vi "DigitalRead.vi"() -> ()   [LabVIEW 2014]
panel:
  in  "Port":u8
  in  "Info In":cluster{"Numeric":u8}
  out "Info Out":cluster{"Numeric":u8}
  out "Reply":string
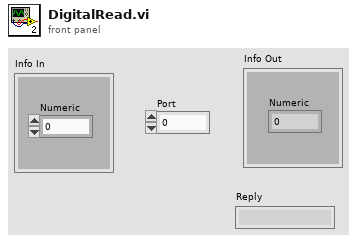
[diagram p1: front panel]
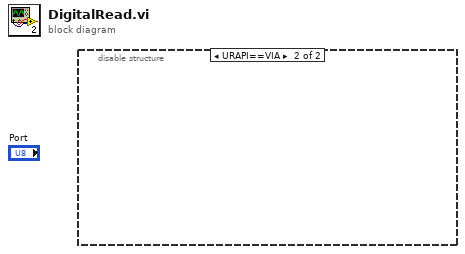
[diagram p0: block diagram]
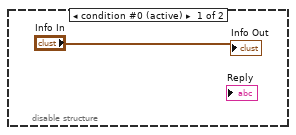
[diagram p2: hidden frame]
diagram:
  n1 = disable-structure shown="URAPI==VIA" {
    frame condition #0 (active) {
      "Info Out" <- "Info In"
    }
    frame condition #1 {
    }
  }
